vi "N8731ACTRL20.vi"() -> ()   [LabVIEW 2017]
uses:
  Controller subVIs/CurrentPSUSettings.vi
  Keysight N8731A conversion/Keysight N8900 Series.lvlib
panel:
  out "time":dbl
  out "I(t)":cluster{dbl[], dbl[]}(graph)
  out "V(t)":cluster{dbl[], dbl[]}(graph)
  in  "Sweep Controller":enum32{"Sweep Mode", "Free Control Mode"}(tab)=enum."Free Control Mode"
  in  "Voltage Limit [V]":dbl=8.0 min=0.0 max=8.0
  in  "Time Delay [s]":dbl=0.15
  in  "Step Size [A]":dbl=5.0 min=0.0 max=400.0
  in  "Start Current [A]":dbl min=0.0 max=400.0
  in  "End Current [A]":dbl=50.0 min=0.0 max=400.0
  out "Approx Sweep Time [min]":dbl
  in  "Start Voltage [V]":dbl min=0.0 max=8.0
  in  "Step Size [mV]":dbl=10.0 min=0.0
  in  "Current Limit [A]":dbl=150.0 min=0.0 max=400.0
  in  "End Voltage[V]":dbl=0.1 min=0.0 max=8.0
  in  "CC(1)/VC(0)":bool
  in  "Time between data points (ms)":i32=500 min=0
  in  "Sweepback Time (s)":dbl min=0.0
  out "Immediate Voltage (V)":dbl
  out "Immediate Current (A)":dbl
  in  "Voltage Set [V]":dbl min=0.0 max=8.0 step=0.001
  in  "Current Set [A]":dbl min=0.0 max=400.0 step=0.1
  out "Status message":string
  in  "Voltmeter channel (6)":i32=6
  in  "em. stop":bool
  in  "Stop Sweep":bool
  out "Voltmeter error message":errorcluster
  in  "Voltmeter Range (V)":dbl caption="0 for Auto range"
  in  "Voltmeter Address (16)":i16=16
  out "PSU error message":errorcluster
  in  "Start Sweep":bool
  in  "Sweepback":bool=TRUE
  in  "Power Output":bool
  in  "OC protection":bool
  in  "OV Value (10V)":dbl=10.0 min=0.5 max=10.0
  out "Sweeping Back":bool
  out "I(V) Graph":cluster{dbl[], dbl[]}(graph)
  in  "VISA resource name":refnum<visa-resource-name>="N8731APSU"
  in  "Filename":string caption="Leave empty to discard data.\nDon't touch during measurement"
  in  "PSU\nVoltage":bool=TRUE caption="Keithley\nVoltage"
  in  "OV protection":bool=TRUE
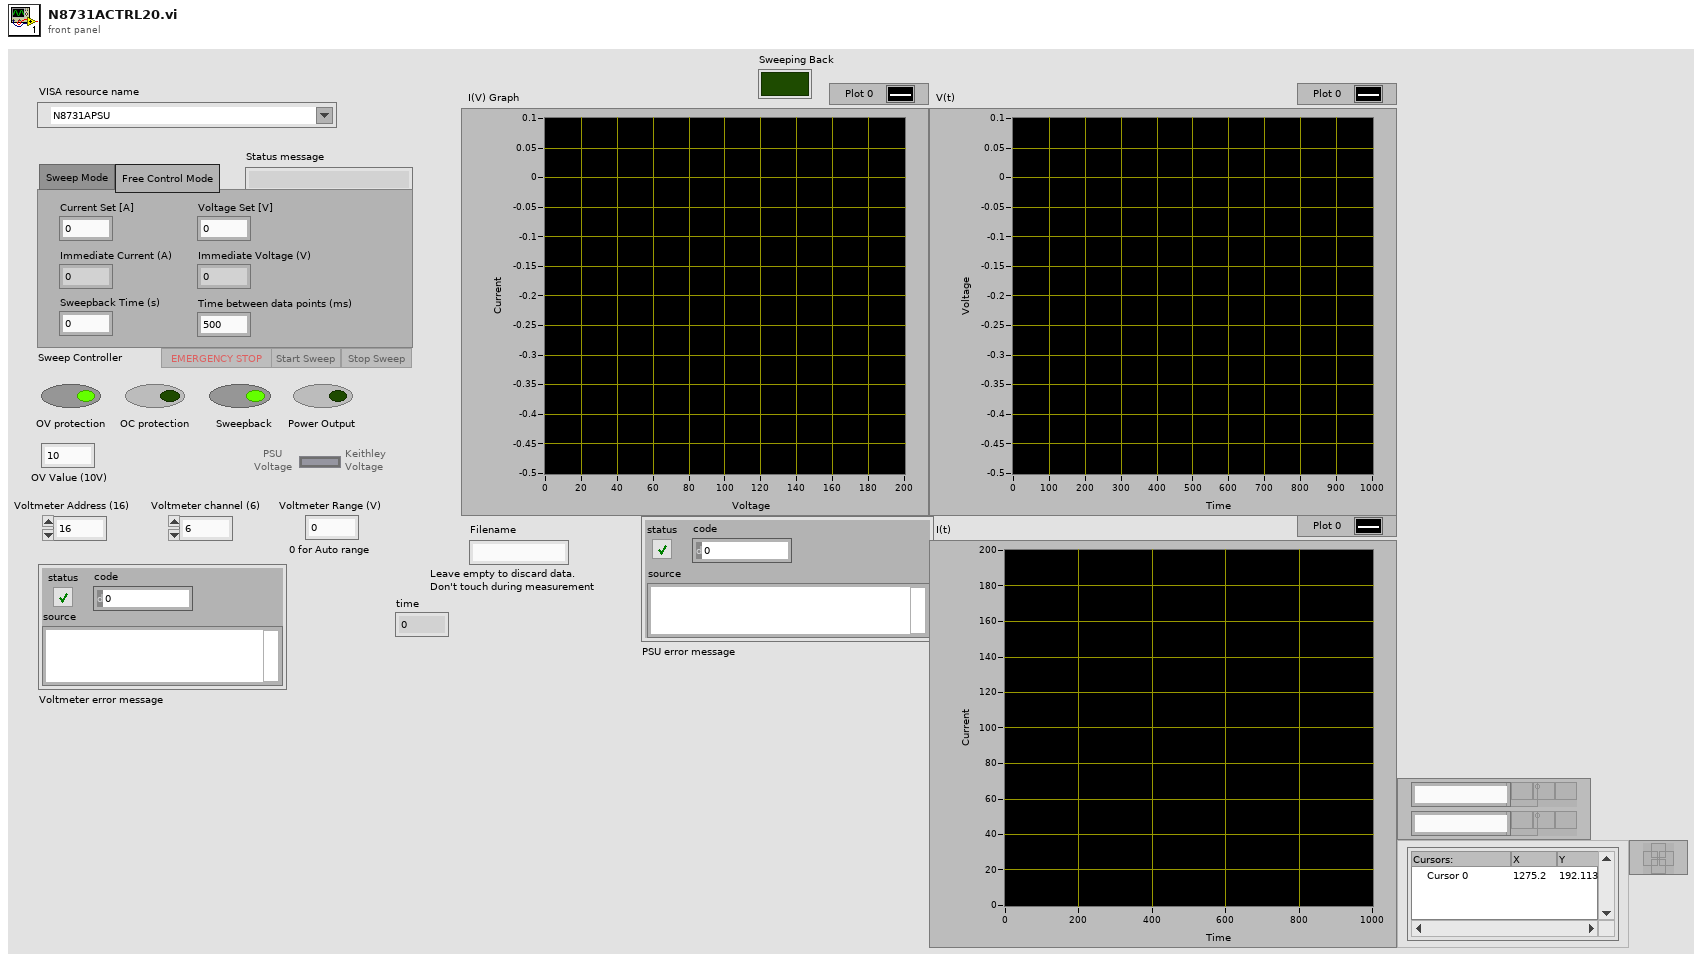
[diagram p1: front panel]
types:
  T1 = enum8{"Enabled", "Disabled", "Disabled and Grayed Out"}
  T2 = cluster{"CC(1)/VC(0)":bool, "Sweep Controller":enum32{"Sweep Mode", "Free Control Mode"}, "   PSU\nVoltage":bool}
  T3 = cluster{"CC(1)/VC(0)":bool, "Sweep Controller":bool, "   PSU\nVoltage":bool}
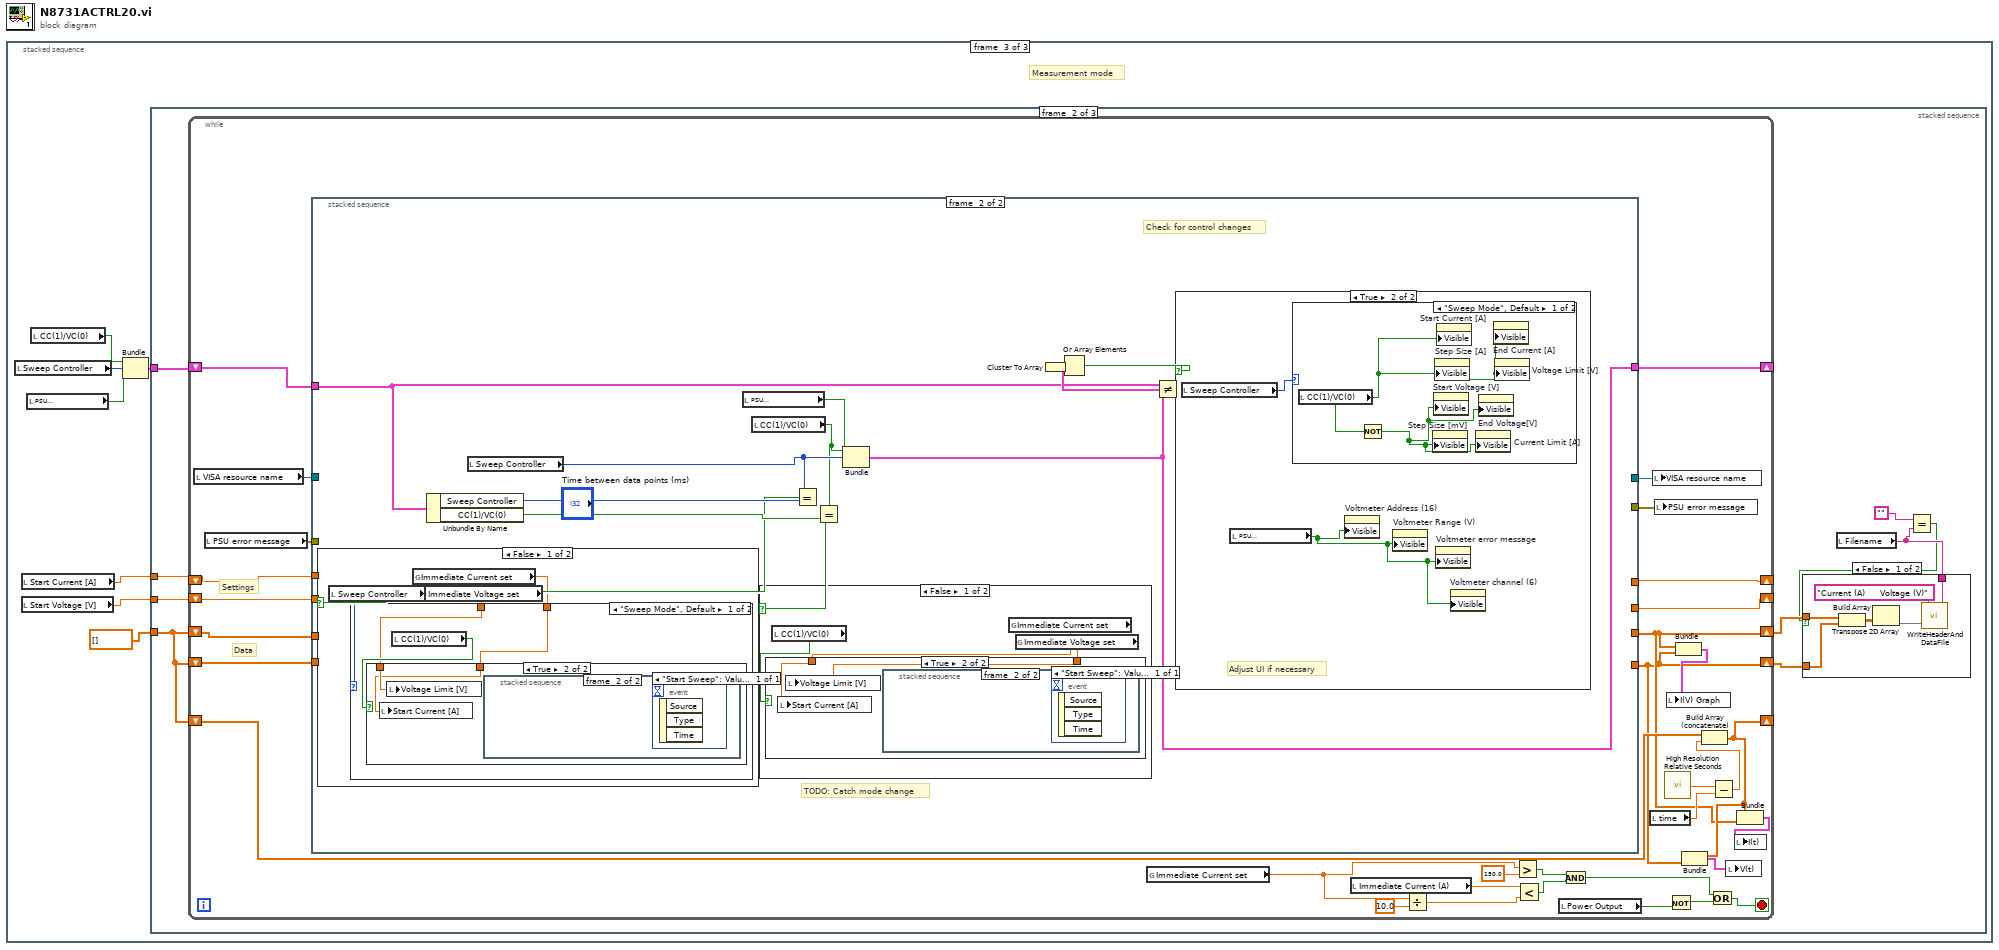
[diagram p0: block diagram]
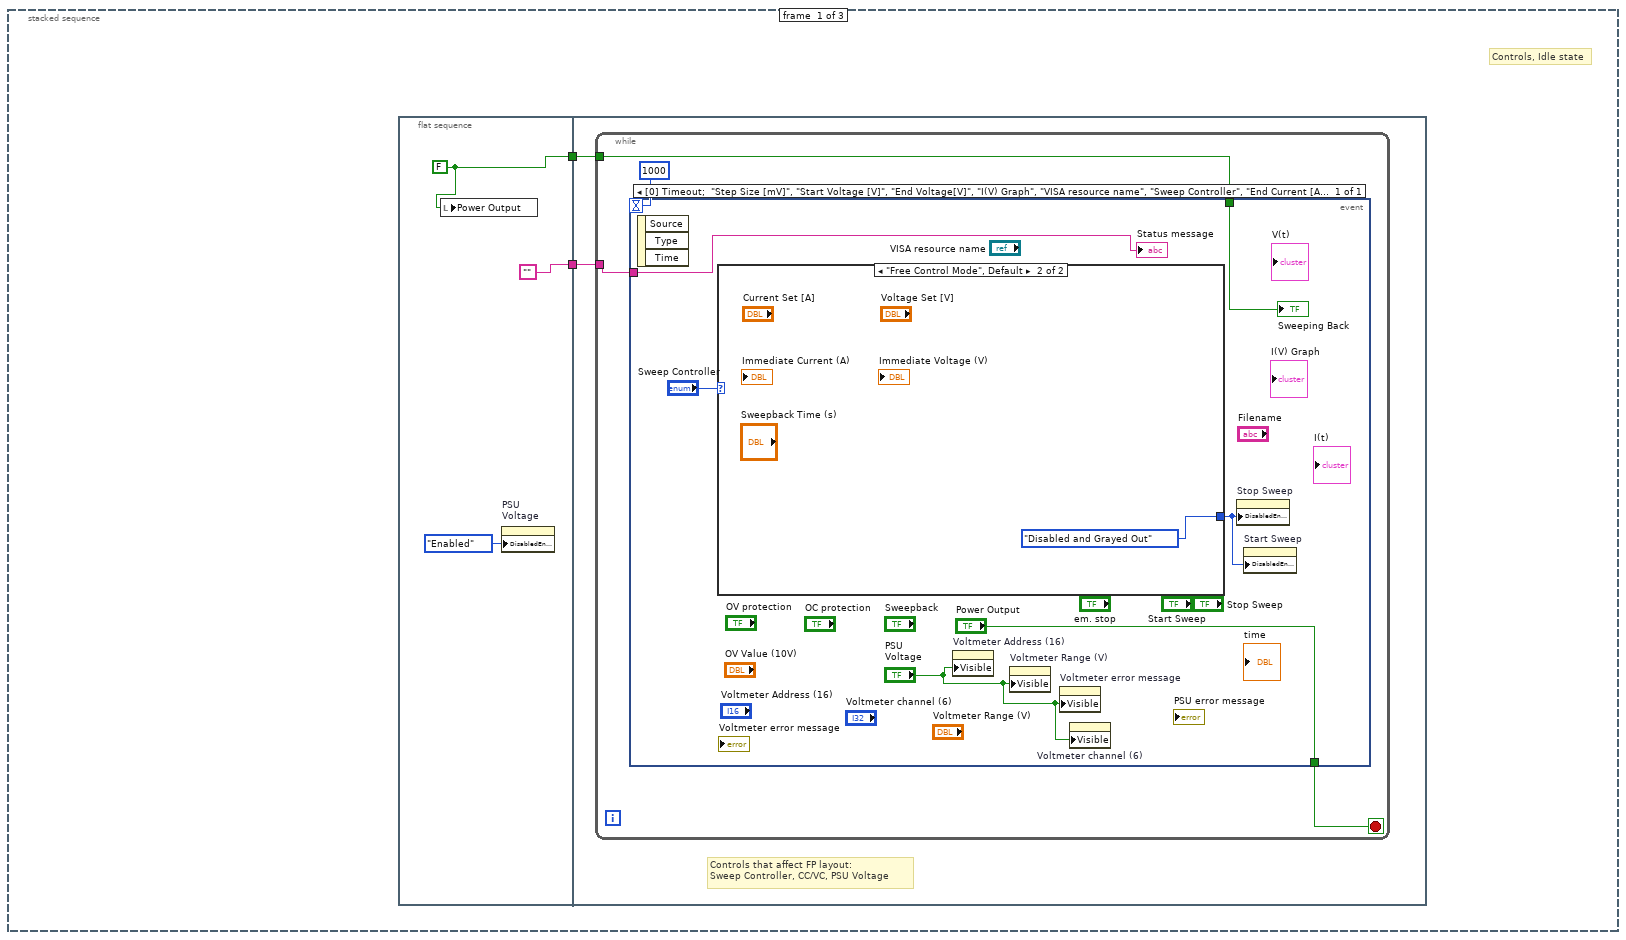
[diagram p2: hidden frame]
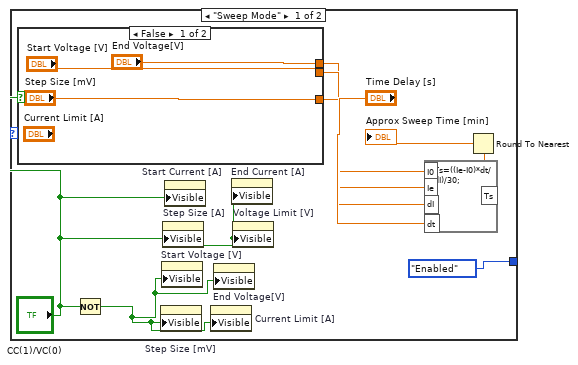
[diagram p3: hidden frame]
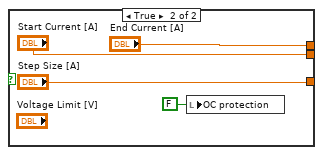
[diagram p4: hidden frame]
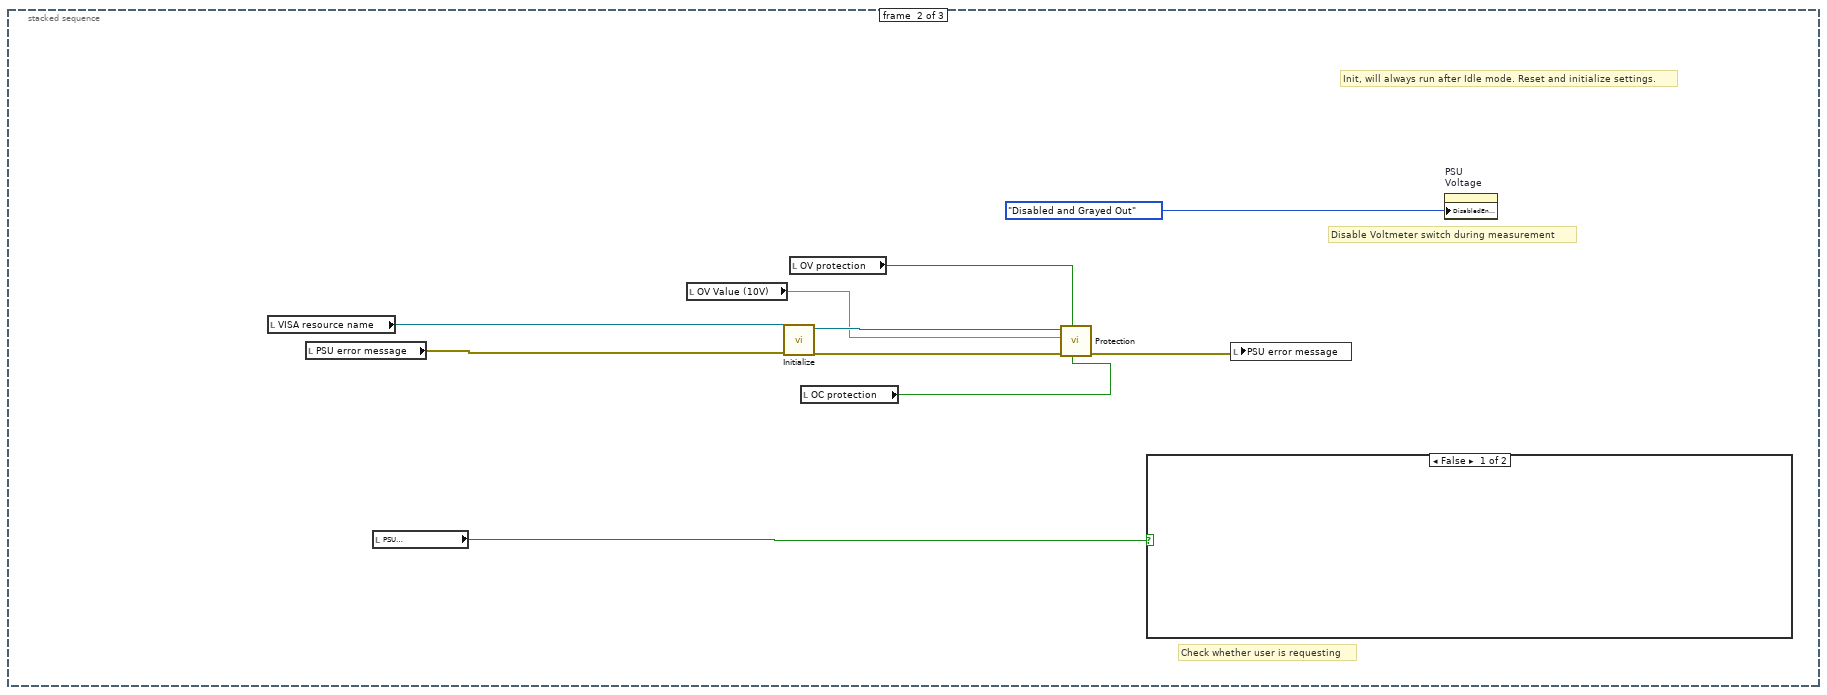
[diagram p5: hidden frame]
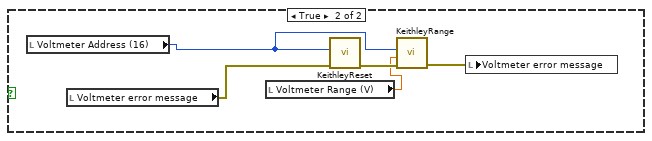
[diagram p6: hidden frame]
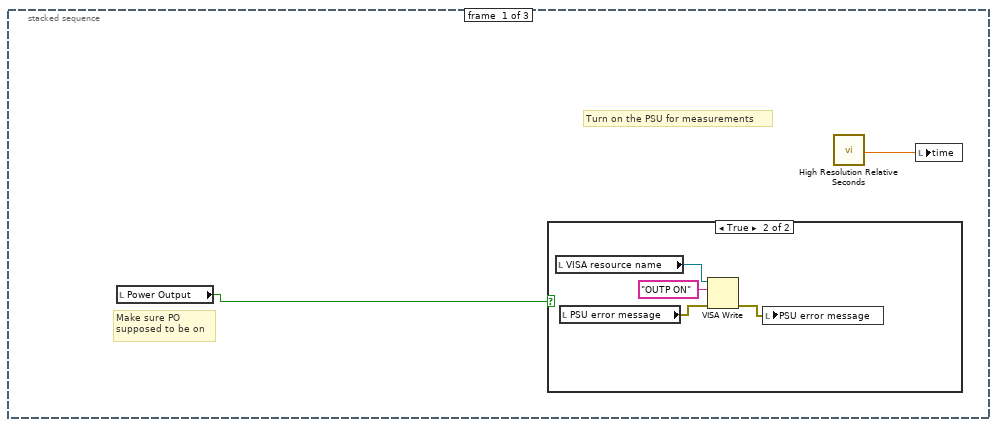
[diagram p7: hidden frame]
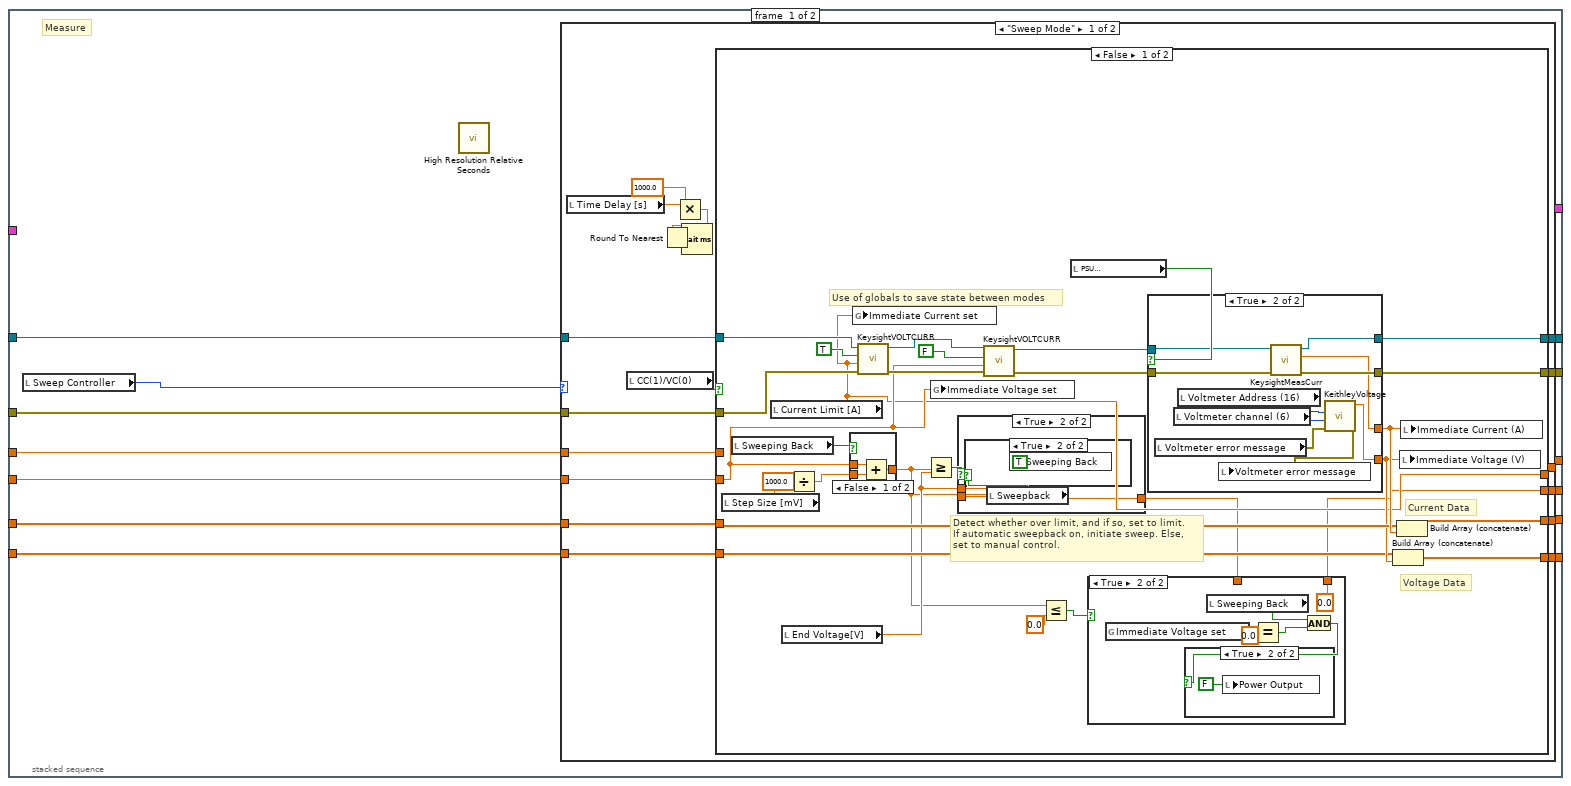
[diagram p10: hidden frame]
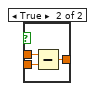
[diagram p13: hidden frame]
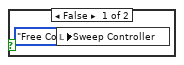
[diagram p15: hidden frame]
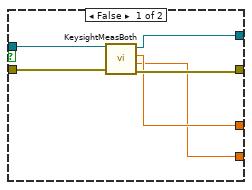
[diagram p16: hidden frame]
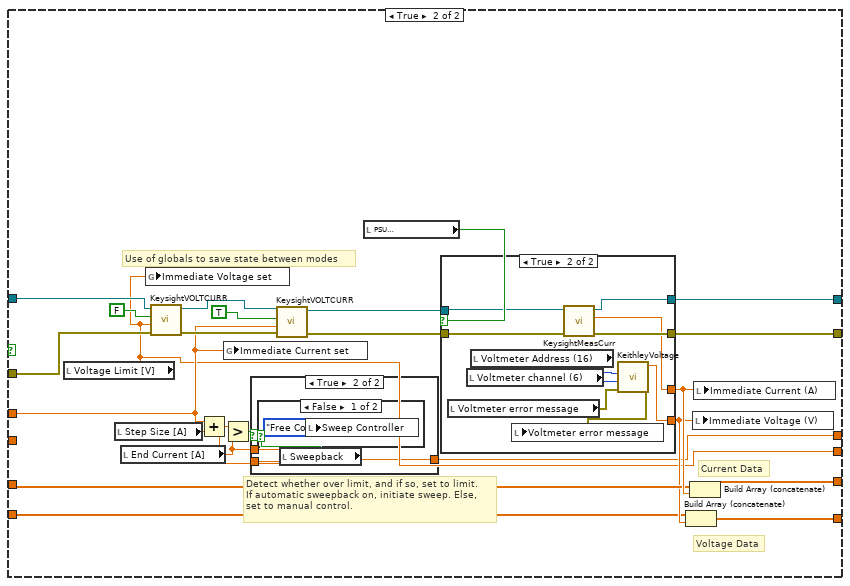
[diagram p17: hidden frame]
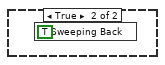
[diagram p19: hidden frame]
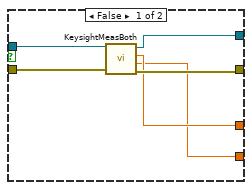
[diagram p20: hidden frame]
diagram:
  n1 = stacked-sequence {
    frame #0 {
      # "Controls, Idle state"
      n2 = flat-sequence {
        tunnel: [w3] -> w2
        tunnel: ["" ("Status message")] -> w1
        tunnel: w2 -> [w7]
        tunnel: w1 -> [w6]
        frame #0 {
          w3 = FALSE ("Sweeping Back")
          n3 = local write "Power Output"(w3) -> ()
          n4 = property on="PSU\nVoltage" class="Bool (strict)"("DisabledEnum"=T1."Enabled" ("Disabled")) -> ()  [unwired: 2 in, 2 out]
        }
        frame #1 {
          # "Controls that affect FP layout:\nSweep Controller, CC/VC, PSU Voltage"
          n5 = while {
            tunnel: w7 -> [w9]
            tunnel: w6 -> [w8]
            stop <- w11 stop-if-true
            n6 = event shown="[0] Timeout;  \"Step Size [mV]\", \"Start Voltage [V]\", \"End Voltage[V]\", \"I(V) Graph\", \"VISA resource name\", \"Sweep Controller\", \"End Current [A]\", \"Stop Sweep\", \"Start Current [A]\", \"Step Size [A]\", \"Time Delay [s]\", \"Current Limit [A]\", \"Voltage Limit [V]\", \"Approx Sweep Time [min]\", \"OV Value (10V)\", \"OC protection\", \"Sweeping Back\", \"Filename\", \"OV protection\", \"PSU Voltage\", \"CC(1)/VC(0)\": Value Change" {
              selector: _ -> [_]
              dyn-events: _ -> [_]
              timeout: 1000 -> [_]
              tunnel: ["Power Output"] -> w11
              tunnel: w9 -> [w14]
              tunnel: w8 -> [w12]
              event Timeout; "Step Size [mV]", "Start Voltage [V]", "End Voltage[V]", "I(V) Graph", "VISA resource name", "Sweep Controller", "End Current [A]", "Stop Sweep", "Start Current [A]", "Step Size [A]", "Time Delay [s]", "Current Limit [A]", "Voltage Limit [V]", "Approx Sweep Time [min]", "OV Value (10V)", "OC protection", "Sweeping Back", "Filename", "OV protection", "PSU\nVoltage", "CC(1)/VC(0)": Value Change {
                n7 = event-data() -> ()  [unwired: 1 in, 3 out]
                n8 = case shown="\"Free Control Mode\", Default" "Sweep Controller" {
                  tunnel: [T1."Enabled" ("Disabled") T1."Disabled and Grayed Out" ("Disabled")] -> w15
                  frame "Sweep Mode" {
                    n9 = case shown="False" "CC(1)/VC(0)" {
                      tunnel: ["Step Size [mV]" "Step Size [A]"] -> w25
                      tunnel: ["Start Voltage [V]" "Start Current [A]"] -> w22
                      tunnel: ["End Voltage[V]" "End Current [A]"] -> w21
                      frame False {
                      }
                      frame True {
                        n10 = local write "OC protection"(FALSE ("OC protection")) -> ()
                      }
                    }
                    n11 = Not(x="CC(1)/VC(0)") -> (.not. x?=w20:bool)
                    n12 = property on="Step Size [mV]" class="DigNum (strict)"("Visible"=w20) -> ()  [unwired: 2 in, 2 out]
                    n13 = property on="Start Voltage [V]" class="DigNum (strict)"("Visible"=w20) -> ()  [unwired: 2 in, 2 out]
                    n14 = property on="Step Size [A]" class="DigNum (strict)"("Visible"="CC(1)/VC(0)") -> ()  [unwired: 2 in, 2 out]
                    n15 = property on="Start Current [A]" class="DigNum (strict)"("Visible"="CC(1)/VC(0)") -> ()  [unwired: 2 in, 2 out]
                    n16 = property on="Current Limit [A]" class="DigNum (strict)"("Visible"=w20) -> ()  [unwired: 2 in, 2 out]
                    n17 = property on="End Voltage[V]" class="DigNum (strict)"("Visible"=w20) -> ()  [unwired: 2 in, 2 out]
                    n18 = property on="End Current [A]" class="DigNum (strict)"("Visible"="CC(1)/VC(0)") -> ()  [unwired: 2 in, 2 out]
                    n19 = property on="Voltage Limit [V]" class="DigNum (strict)"("Visible"="CC(1)/VC(0)") -> ()  [unwired: 2 in, 2 out]
                    n20 = formula code="Ts=((Ie-I0)*dt/dI)/30;"("I0"=w22, "Ie"=w21, "dI"=w25, "dt"="Time Delay [s]") -> ("Ts"=w24:dbl)
                    n21 = Round To Nearest(number=w24) -> (nearest integer value=→"Approx Sweep Time [min]":dbl)
                  }
                  frame "Free Control Mode", Default {
                  }
                }
                n22 = property on="Voltmeter Address (16)" class="DigNum (strict)"("Visible"="PSU\nVoltage") -> ()  [unwired: 2 in, 2 out]
                n23 = property on="Voltmeter Range (V)" class="DigNum (strict)"("Visible"="PSU\nVoltage") -> ()  [unwired: 2 in, 2 out]
                n24 = property on="Voltmeter error message" class="Clust (strict)"("Visible"="PSU\nVoltage") -> ()  [unwired: 2 in, 2 out]
                n25 = property on="Voltmeter channel (6)" class="DigNum (strict)"("Visible"="PSU\nVoltage") -> ()  [unwired: 2 in, 2 out]
                n26 = property on="Stop Sweep" class="Bool"("DisabledEnum"=w15) -> ()  [unwired: 2 in, 2 out]
                n27 = property on="Start Sweep" class="Bool"("DisabledEnum"=w15) -> ()  [unwired: 2 in, 2 out]
                "Sweeping Back" <- w14
                "Status message" <- w12
              }
            }
          }
        }
      }
    }
    frame #1 {
      # "Check whether user is requesting"
      # "Disable Voltmeter switch during measurement"
      # "Init, will always run after Idle mode. Reset and initialize settings."
      n28 = local read "VISA resource name"() -> (w42:refnum<visa-resource-name>)
      n29 = local read "PSU error message"() -> (w37:errorcluster)
      n30 = local read "PSU\nVoltage"() -> (w36:bool)
      n31 = local read "OV Value (10V)"() -> (w41:dbl)
      n32 = call "Initialize.vi"("error in (no error)"=w37, "VISA resource name"=w42) -> ("error out"=w43:errorcluster, "VISA resource name out"=w44:refnum<visa-resource-name>)  [unwired: 8 in]
      n33 = local read "OV protection"() -> (w39:bool)
      n34 = local read "OC protection"() -> (w40:bool)
      n35 = call "Protection.vi"("OC protection"=w40, "OV protection"=w39, "error in (no error)"=w43, "OV Value (10V)"=w41, "VISA resource name"=w44) -> ("error out"=w38:errorcluster)  [unwired: 5 in, 1 out]
      n36 = case shown="False" w36 {
        frame False {
        }
        frame True {
          n37 = local read "Voltmeter Address (16)"() -> (w45:i16)
          n38 = local read "Voltmeter error message"() -> (w47:errorcluster)
          n39 = local read "Voltmeter Range (V)"() -> (w46:dbl)
          n40 = call "KeithleyReset.vi"("error in"=w47, "address (16)"=w45) -> ("error out"=w48:errorcluster)  [unwired: 9 in]
          n41 = call "KeithleyRange.vi"("error in"=w48, "Range (V)/Auto(0)"=w46, "address (16)"=w45) -> ("error out"=w49:errorcluster)  [unwired: 8 in]
          n42 = local write "Voltmeter error message"(w49) -> ()
        }
      }
      n43 = local write "PSU error message"(w38) -> ()
      n44 = property on="PSU\nVoltage" class="Bool (strict)"("DisabledEnum"=T1."Disabled and Grayed Out" ("Disabled")) -> ()  [unwired: 2 in, 2 out]
    }
    frame #2 {
      # "Measurement mode"
      n45 = local read "Sweep Controller"() -> (w55:enum32{"Sweep Mode", "Free Control Mode"})
      n46 = local read "Start Current [A]"() -> (w52:dbl)
      n47 = local read "Start Voltage [V]"() -> (w51:dbl)
      n48 = local read "PSU\nVoltage"() -> (w54:bool)
      n49 = local read "CC(1)/VC(0)"() -> (w56:bool)
      n50 = Bundle("CC(1)/VC(0)"=w56, "Sweep Controller"=w55, "PSU\nVoltage"=w54) -> (w53:T2)  [unwired: 1 in]
      n51 = stacked-sequence {
        tunnel: w53 -> [_ w71 _]
        tunnel: w52 -> [_ w70 _]
        tunnel: w51 -> [_ w69 _]
        tunnel: dbl[] [] -> [_ w63 _]
        frame #0 {
          # "Make sure PO\nsupposed to be on"
          # "Turn on the PSU for measurements"
          n52 = local read "Power Output"() -> (w58:bool)
          n53 = case shown="True" w58 {
            frame False {
            }
            frame True {
              n54 = local read "VISA resource name"() -> (w61:refnum<visa-resource-name>)
              n55 = local read "PSU error message"() -> (w60:errorcluster)
              n56 = VISA Write(VISA resource name=w61, write buffer="OUTP ON", error in (no error)=w60) -> (error out=w59:errorcluster)  [unwired: 2 out]
              n57 = local write "PSU error message"(w59) -> ()
            }
          }
          n58 = call <vilib>:"High Resolution Relative Seconds.vi"() -> ("relative seconds"=w57:dbl)
          n59 = local write "time"(w57) -> ()
        }
        frame #1 {
          n60 = while {
            shift-right: [w109] -> _
            shift-left: w71 -> [w110]
            shift-right: [w100] -> _
            shift-left: w69 -> [w98]
            shift-right: [w101] -> _
            shift-left: w70 -> [w106]
            shift-right: [w91] -> w68
            shift-left: w63 -> [w103]
            shift-right: [w90] -> w67
            shift-left: w63 -> [w102]
            shift-right: [w92] -> _
            shift-left: w63 -> [w96]
            stop <- w78 stop-if-true
            # "Data"
            # "Settings"
            n61 = local read "VISA resource name"() -> (w108:refnum<visa-resource-name>)
            n62 = local read "PSU error message"() -> (w107:errorcluster)
            n63 = stacked-sequence {
              tunnel: w110 -> [_ w295]
              tunnel: [_ w299] -> w109
              tunnel: w108 -> [w122 _]
              tunnel: w107 -> [w121 _]
              tunnel: w106 -> [w120 _]
              tunnel: [w119 _] -> w105
              tunnel: [w118 _] -> w104
              tunnel: w103 -> [w117 _]
              tunnel: [w116 _] -> w91
              tunnel: w102 -> [w115 _]
              tunnel: [w114 _] -> w90
              tunnel: [w113 _] -> w101
              tunnel: [w112 _] -> w100
              tunnel: w98 -> [w111 _]
              frame #0 {
                # "Measure"
                n64 = local read "Sweep Controller"() -> (w123:enum32{"Sweep Mode", "Free Control Mode"})
                n65 = call <vilib>:"High Resolution Relative Seconds.vi"() -> ()  [unwired: 1 out]
                n66 = case shown="\"Sweep Mode\"" w123 {
                  tunnel: w122 -> [w139 w272]
                  tunnel: w121 -> [w138 w271]
                  tunnel: w120 -> [w137 _]
                  tunnel: [w136 w270] -> w119
                  tunnel: [w135 w269] -> w118
                  tunnel: w117 -> [w134 w268]
                  tunnel: [w133 w267] -> w116
                  tunnel: w115 -> [w132 w266]
                  tunnel: [w131 w265] -> w114
                  tunnel: [w130 w253] -> w113
                  tunnel: [w129 w252] -> w112
                  tunnel: w111 -> [w128 _]
                  frame "Sweep Mode" {
                    n67 = local read "Time Delay [s]"() -> (w127:dbl)
                    n68 = local read "CC(1)/VC(0)"() -> (w140:bool)
                    n69 = Multiply(x=w127, y=1000.0) -> (x*y=w125:dbl)
                    n70 = Round To Nearest(number=w125) -> (nearest integer value=w124:dbl)
                    n71 = Wait (ms)(milliseconds to wait=w124) -> ()  [unwired: 1 out]
                    n72 = case shown="False" w140 {
                      tunnel: w139 -> [w166 w225]
                      tunnel: w138 -> [w165 w224]
                      tunnel: w137 -> [_ w223]
                      tunnel: [w161 w218] -> w136
                      tunnel: [w160 w217] -> w135
                      tunnel: w134 -> [w158 w215]
                      tunnel: [w149 w214] -> w133
                      tunnel: w132 -> [w156 w212]
                      tunnel: [w155 w211] -> w131
                      tunnel: [w148 w209] -> w130
                      tunnel: [w142 w210] -> w129
                      tunnel: w128 -> [w150 _]
                      frame False {
                        # "Use of globals to save state between modes"
                        # "Detect whether over limit, and if so, set to limit.\nIf automatic sweepback on, initiate sweep. Else,\nset to manual control."
                        # "Voltage Data"
                        # "Current Data"
                        n73 = local read "Step Size [mV]"() -> (w153:dbl)
                        n74 = local read "Sweeping Back"() -> (w146:bool)
                        n75 = local read "Current Limit [A]"() -> (w148:dbl)
                        n76 = local read "End Voltage[V]"() -> (w147:dbl)
                        n77 = Divide(x=w153, y=1000.0) -> (x/y=w152:dbl)
                        n78 = case shown="False" w146 {
                          tunnel: [w181 w182] -> w144
                          tunnel: w152 -> [w180 w184]
                          tunnel: w150 -> [w179 w183]
                          frame False {
                            n79 = Add(x=w179, y=w180) -> (x+y=w181:dbl)
                          }
                          frame True {
                            n80 = Subtract(x=w183, y=w184) -> (x-y=w182:dbl)
                          }
                        }
                        n81 = global write "CurrentPSUSettings.vi" "Immediate Current set"(w148) -> ()
                        n82 = call "KeysightVOLTCURR.vi"("error in (no error)"=w165, "CURR/VOLT (A/V)"=w148, "CURR (1)/VOLT (0)"=TRUE, "VISA resource name"=w166) -> ("error out"=w167:errorcluster, "VISA resource name out"=w168:refnum<visa-resource-name>)  [unwired: 6 in]
                        n83 = Greater Or Equal?(x=w144, y=w147) -> (x >= y?=w154:bool)
                        n84 = global write "CurrentPSUSettings.vi" "Immediate Voltage set"(w150) -> ()
                        n85 = case shown="True" w154 {
                          tunnel: w144 -> [w185 _]
                          tunnel: [w185 w187] -> w143
                          tunnel: w147 -> [_ w187]
                          frame False {
                          }
                          frame True {
                            n86 = local read "Sweepback"() -> (w186:bool)
                            n87 = case shown="True" w186 {
                              frame False {
                                n88 = local write "Sweep Controller"(enum32{"Sweep Mode", "Free Control Mode"}."Free Control Mode" ("Sweep Controller")) -> ()
                              }
                              frame True {
                                n89 = local write "Sweeping Back"(TRUE ("Sweeping Back")) -> ()
                              }
                            }
                          }
                        }
                        n90 = call "KeysightVOLTCURR.vi"("error in (no error)"=w167, "CURR/VOLT (A/V)"=w150, "CURR (1)/VOLT (0)"=FALSE, "VISA resource name"=w168) -> ("error out"=w162:errorcluster, "VISA resource name out"=w163:refnum<visa-resource-name>)  [unwired: 6 in]
                        n91 = Less Or Equal?(x=w144, y=0.0) -> (x <= y?=w141:bool)
                        n92 = local read "PSU\nVoltage"() -> (w164:bool)
                        n93 = case shown="True" w141 {
                          tunnel: w143 -> [w171 _]
                          tunnel: [w171 0.0 ("End Voltage[V]")] -> w142
                          frame False {
                          }
                          frame True {
                            n94 = global read "CurrentPSUSettings.vi" "Immediate Voltage set"() -> (w175:dbl)
                            n95 = local read "Sweeping Back"() -> (w176:bool)
                            n96 = Equal?(x=w175, y=0.0) -> (x = y?=w173:bool)
                            n97 = And(x=w176, y=w173) -> (x .and. y?=w172:bool)
                            n98 = case shown="True" w172 {
                              frame False {
                              }
                              frame True {
                                n99 = local write "Power Output"(FALSE ("Power Output")) -> ()
                              }
                            }
                          }
                        }
                        n100 = case shown="True" w164 {
                          tunnel: w163 -> [w195 w205]
                          tunnel: w162 -> [w194 w204]
                          tunnel: [w193 w199] -> w161
                          tunnel: [w192 w198] -> w160
                          tunnel: [w191 w197] -> w159
                          tunnel: [w190 w196] -> w157
                          frame False {
                            n101 = call "KeysightMeasBoth.vi"("error in (no error)"=w194, "VISA resource name"=w195) -> ("error out"=w192:errorcluster, "VOLT"=w190:dbl, "CURR"=w191:dbl, "VISA resource name out"=w193:refnum<visa-resource-name>)  [unwired: 6 in]
                          }
                          frame True {
                            n102 = local read "Voltmeter error message"() -> (w201:errorcluster)
                            n103 = local read "Voltmeter channel (6)"() -> (w203:i32)
                            n104 = local read "Voltmeter Address (16)"() -> (w202:i16)
                            n105 = call "KeysightMeasCurr.vi"("error in (no error)"=w204, "VISA resource name"=w205) -> ("error out"=w198:errorcluster, "CURR"=w197:dbl, "VISA resource name out"=w199:refnum<visa-resource-name>)  [unwired: 7 in]
                            n106 = call "KeithleyVoltage.vi"("error in"=w201, "channel (6)"=w203, "address (16)"=w202) -> ("error out"=w200:errorcluster, "Voltage"=w196:dbl)  [unwired: 7 in]
                            n107 = local write "Voltmeter error message"(w200) -> ()
                          }
                        }
                        n108 = Build Array (concatenate)(w156, w157) -> (w155:dbl[])
                        n109 = Build Array (concatenate)(w158, w159) -> (w149:dbl[])
                        n110 = local write "Immediate Voltage (V)"(w157) -> ()
                        n111 = local write "Immediate Current (A)"(w159) -> ()
                      }
                      frame True {
                        # "Use of globals to save state between modes"
                        # "Detect whether over limit, and if so, set to limit.\nIf automatic sweepback on, initiate sweep. Else,\nset to manual control."
                        # "Voltage Data"
                        # "Current Data"
                        n112 = local read "Voltage Limit [V]"() -> (w210:dbl)
                        n113 = local read "Step Size [A]"() -> (w222:dbl)
                        n114 = local read "End Current [A]"() -> (w206:dbl)
                        n115 = global write "CurrentPSUSettings.vi" "Immediate Voltage set"(w210) -> ()
                        n116 = call "KeysightVOLTCURR.vi"("error in (no error)"=w224, "CURR/VOLT (A/V)"=w210, "CURR (1)/VOLT (0)"=FALSE, "VISA resource name"=w225) -> ("error out"=w226:errorcluster, "VISA resource name out"=w227:refnum<visa-resource-name>)  [unwired: 6 in]
                        n117 = Add(x=w223, y=w222) -> (x+y=w207:dbl)
                        n118 = Greater?(x=w207, y=w206) -> (0:w208:bool)
                        n119 = global write "CurrentPSUSettings.vi" "Immediate Current set"(w223) -> ()
                        n120 = case shown="True" w208 {
                          tunnel: w207 -> [w230 _]
                          tunnel: [w230 w232] -> w209
                          tunnel: w206 -> [_ w232]
                          frame False {
                          }
                          frame True {
                            n121 = local read "Sweepback"() -> (w231:bool)
                            n122 = case shown="False" w231 {
                              frame False {
                                n123 = local write "Sweep Controller"(enum32{"Sweep Mode", "Free Control Mode"}."Free Control Mode" ("Sweep Controller")) -> ()
                              }
                              frame True {
                                n124 = local write "Sweeping Back"(TRUE ("Sweeping Back")) -> ()
                              }
                            }
                          }
                        }
                        n125 = call "KeysightVOLTCURR.vi"("error in (no error)"=w226, "CURR/VOLT (A/V)"=w223, "CURR (1)/VOLT (0)"=TRUE, "VISA resource name"=w227) -> ("error out"=w219:errorcluster, "VISA resource name out"=w220:refnum<visa-resource-name>)  [unwired: 6 in]
                        n126 = local read "PSU\nVoltage"() -> (w221:bool)
                        n127 = case shown="True" w221 {
                          tunnel: w220 -> [w240 w250]
                          tunnel: w219 -> [w239 w249]
                          tunnel: [w238 w244] -> w218
                          tunnel: [w237 w243] -> w217
                          tunnel: [w236 w242] -> w216
                          tunnel: [w235 w241] -> w213
                          frame False {
                            n128 = call "KeysightMeasBoth.vi"("error in (no error)"=w239, "VISA resource name"=w240) -> ("error out"=w237:errorcluster, "VOLT"=w235:dbl, "CURR"=w236:dbl, "VISA resource name out"=w238:refnum<visa-resource-name>)  [unwired: 6 in]
                          }
                          frame True {
                            n129 = local read "Voltmeter error message"() -> (w246:errorcluster)
                            n130 = local read "Voltmeter channel (6)"() -> (w248:i32)
                            n131 = local read "Voltmeter Address (16)"() -> (w247:i16)
                            n132 = call "KeysightMeasCurr.vi"("error in (no error)"=w249, "VISA resource name"=w250) -> ("error out"=w243:errorcluster, "CURR"=w242:dbl, "VISA resource name out"=w244:refnum<visa-resource-name>)  [unwired: 7 in]
                            n133 = call "KeithleyVoltage.vi"("error in"=w246, "channel (6)"=w248, "address (16)"=w247) -> ("error out"=w245:errorcluster, "Voltage"=w241:dbl)  [unwired: 7 in]
                            n134 = local write "Voltmeter error message"(w245) -> ()
                          }
                        }
                        n135 = Build Array (concatenate)(w212, w213) -> (w211:dbl[])
                        n136 = Build Array (concatenate)(w215, w216) -> (w214:dbl[])
                        n137 = local write "Immediate Voltage (V)"(w213) -> ()
                        n138 = local write "Immediate Current (A)"(w216) -> ()
                      }
                    }
                  }
                  frame "Free Control Mode", Default {
                    # "Use of globals to save state between modes"
                    # "Detect whether over limit, and if so, set to limit.\nIf automatic sweepback on, initiate sweep. Else,\nset to manual control."
                    # "Voltage Data"
                    # "Current Data"
                    n139 = local read "Time between data points (ms)"() -> (w251:i32)
                    n140 = local read "Current Set [A]"() -> (w264:dbl)
                    n141 = Wait (ms)(milliseconds to wait=w251) -> ()  [unwired: 1 out]
                    n142 = local read "Voltage Set [V]"() -> (w255:dbl)
                    n143 = global write "CurrentPSUSettings.vi" "Immediate Current set"(w264) -> ()
                    n144 = call "KeysightVOLTCURR.vi"("error in (no error)"=w271, "CURR/VOLT (A/V)"=w264, "CURR (1)/VOLT (0)"=TRUE, "VISA resource name"=w272) -> ("error out"=w260:errorcluster, "VISA resource name out"=w261:refnum<visa-resource-name>)  [unwired: 6 in]
                    n145 = global write "CurrentPSUSettings.vi" "Immediate Voltage set"(w255) -> ()
                    n146 = call "KeysightVOLTCURR.vi"("error in (no error)"=w260, "CURR/VOLT (A/V)"=w255, "CURR (1)/VOLT (0)"=FALSE, "VISA resource name"=w261) -> ("error out"=w257:errorcluster, "VISA resource name out"=w258:refnum<visa-resource-name>)  [unwired: 6 in]
                    n147 = local read "PSU\nVoltage"() -> (w259:bool)
                    n148 = case shown="True" w259 {
                      tunnel: w258 -> [w278 w288]
                      tunnel: w257 -> [w277 w287]
                      tunnel: [w276 w282] -> w270
                      tunnel: [w275 w281] -> w269
                      tunnel: [w274 w280] -> w256
                      tunnel: [w273 w279] -> w254
                      frame False {
                        n149 = call "KeysightMeasBoth.vi"("error in (no error)"=w277, "VISA resource name"=w278) -> ("error out"=w275:errorcluster, "VOLT"=w273:dbl, "CURR"=w274:dbl, "VISA resource name out"=w276:refnum<visa-resource-name>)  [unwired: 6 in]
                      }
                      frame True {
                        n150 = local read "Voltmeter error message"() -> (w284:errorcluster)
                        n151 = local read "Voltmeter channel (6)"() -> (w286:i32)
                        n152 = local read "Voltmeter Address (16)"() -> (w285:i16)
                        n153 = call "KeysightMeasCurr.vi"("error in (no error)"=w287, "VISA resource name"=w288) -> ("error out"=w281:errorcluster, "CURR"=w280:dbl, "VISA resource name out"=w282:refnum<visa-resource-name>)  [unwired: 7 in]
                        n154 = call "KeithleyVoltage.vi"("error in"=w284, "channel (6)"=w286, "address (16)"=w285) -> ("error out"=w283:errorcluster, "Voltage"=w279:dbl)  [unwired: 7 in]
                        n155 = local write "Voltmeter error message"(w283) -> ()
                      }
                    }
                    n156 = local write "Immediate Voltage (V)"(w254) -> ()
                    n157 = Build Array (concatenate)(w266, w254) -> (w265:dbl[])
                    n158 = global read "CurrentPSUSettings.vi" "Immediate Current set"() -> (w253:dbl)
                    n159 = global read "CurrentPSUSettings.vi" "Immediate Voltage set"() -> (w252:dbl)
                    n160 = Build Array (concatenate)(w268, w256) -> (w267:dbl[])
                    n161 = local write "Immediate Current (A)"(w256) -> ()
                  }
                }
              }
              frame #1 {
                # "TODO: Catch mode change"
                # "Check for control changes"
                n162 = Unbundle By Name(w295) -> ("Sweep Controller"=w293:enum32{"Sweep Mode", "Free Control Mode"}, "CC(1)/VC(0)"=w292:bool)
                n163 = local read "Sweep Controller"() -> (w294:enum32{"Sweep Mode", "Free Control Mode"})
                n164 = local read "PSU\nVoltage"() -> (w300:bool)
                n165 = local read "CC(1)/VC(0)"() -> (w291:bool)
                n166 = Equal?(x=w294, y=w293) -> (x = y?=w290:bool)
                n167 = case shown="False" w290 {
                  frame False {
                    n168 = local read "Sweep Controller"() -> (w312:enum32{"Sweep Mode", "Free Control Mode"})
                    n169 = global read "CurrentPSUSettings.vi" "Immediate Current set"() -> (w310:dbl)
                    n170 = global read "CurrentPSUSettings.vi" "Immediate Voltage set"() -> (w311:dbl)
                    n171 = case shown="\"Sweep Mode\", Default" w312 {
                      tunnel: w311 -> [w314 w323]
                      tunnel: w310 -> [w313 w322]
                      frame "Sweep Mode", Default {
                        n172 = local read "CC(1)/VC(0)"() -> (w315:bool)
                        n173 = case shown="True" w315 {
                          tunnel: w314 -> [w317 w320]
                          tunnel: w313 -> [w316 w319]
                          frame False {
                            n174 = local write "Start Voltage [V]"(w317) -> ()
                            n175 = local write "Current Limit [A]"(w316) -> ()
                            n176 = stacked-sequence {
                              frame #0 {
                                n177 = local write "Status message"("Awaiting sweep confirmation" ("Status message")) -> ()
                              }
                              frame #1 {
                                n178 = event shown="[0] \"Start Sweep\": Value Change" {
                                selector: _ -> [_]
                                dyn-events: _ -> [_]
                                timeout: _ -> [_]
                                event "Start Sweep": Value Change {
                                n179 = event-data() -> ()  [unwired: 1 in, 3 out]
                                }
                                }
                              }
                            }
                          }
                          frame True {
                            n180 = local write "Start Current [A]"(w319) -> ()
                            n181 = local write "Voltage Limit [V]"(w320) -> ()
                            n182 = stacked-sequence {
                              frame #0 {
                                n183 = local write "Status message"("Awaiting sweep confirmation" ("Status message")) -> ()
                              }
                              frame #1 {
                                n184 = event shown="[0] \"Start Sweep\": Value Change" {
                                selector: _ -> [_]
                                dyn-events: _ -> [_]
                                timeout: _ -> [_]
                                event "Start Sweep": Value Change {
                                n185 = event-data() -> ()  [unwired: 1 in, 3 out]
                                }
                                }
                              }
                            }
                          }
                        }
                      }
                      frame "Free Control Mode" {
                        n186 = local write "Voltage Set [V]"(w323) -> ()
                        n187 = local write "Current Set [A]"(w322) -> ()
                      }
                    }
                  }
                  frame True {
                  }
                }
                n188 = Equal?(x=w291, y=w292) -> (x = y?=w289:bool)
                n189 = case shown="False" w289 {
                  frame False {
                    n190 = local read "CC(1)/VC(0)"() -> (w303:bool)
                    n191 = global read "CurrentPSUSettings.vi" "Immediate Current set"() -> (w301:dbl)
                    n192 = global read "CurrentPSUSettings.vi" "Immediate Voltage set"() -> (w302:dbl)
                    n193 = case shown="True" w303 {
                      tunnel: w302 -> [w305 w308]
                      tunnel: w301 -> [w304 w307]
                      frame False {
                        n194 = local write "Start Voltage [V]"(w305) -> ()
                        n195 = local write "Current Limit [A]"(w304) -> ()
                        n196 = stacked-sequence {
                          frame #0 {
                            n197 = local write "Status message"("Awaiting sweep confirmation" ("Status message")) -> ()
                          }
                          frame #1 {
                            n198 = event shown="[0] \"Start Sweep\": Value Change" {
                              selector: _ -> [_]
                              dyn-events: _ -> [_]
                              timeout: _ -> [_]
                              event "Start Sweep": Value Change {
                                n199 = event-data() -> ()  [unwired: 1 in, 3 out]
                              }
                            }
                          }
                        }
                      }
                      frame True {
                        n200 = local write "Start Current [A]"(w307) -> ()
                        n201 = local write "Voltage Limit [V]"(w308) -> ()
                        n202 = stacked-sequence {
                          frame #0 {
                            n203 = local write "Status message"("Awaiting sweep confirmation" ("Status message")) -> ()
                          }
                          frame #1 {
                            n204 = event shown="[0] \"Start Sweep\": Value Change" {
                              selector: _ -> [_]
                              dyn-events: _ -> [_]
                              timeout: _ -> [_]
                              event "Start Sweep": Value Change {
                                n205 = event-data() -> ()  [unwired: 1 in, 3 out]
                              }
                            }
                          }
                        }
                      }
                    }
                  }
                  frame True {
                  }
                }
                n206 = Bundle("CC(1)/VC(0)"=w291, "Sweep Controller"=w294, "PSU\nVoltage"=w300) -> (w299:T2)  [unwired: 1 in]
                n207 = Not Equal?(x=w295, y=w299) -> (x != y?=w298:T3)
                n208 = Cluster To Array(cluster=w298) -> (array=w297:bool[])
                n209 = Or Array Elements(Boolean array=w297) -> (logical OR=w296:bool)
                n210 = case shown="True" w296 {
                  frame False {
                  }
                  frame True {
                    # "Adjust UI if necessary"
                    n211 = local read "Sweep Controller"() -> (w325:enum32{"Sweep Mode", "Free Control Mode"})
                    n212 = local read "PSU\nVoltage"() -> (w324:bool)
                    n213 = case shown="\"Sweep Mode\", Default" w325 {
                      frame "Sweep Mode", Default {
                        n214 = local read "CC(1)/VC(0)"() -> (w326:bool)
                        n215 = Not(x=w326) -> (.not. x?=w327:bool)
                        n216 = property on="Step Size [mV]" class="DigNum (strict)"("Visible"=w327) -> ()  [unwired: 2 in, 2 out]
                        n217 = property on="Start Voltage [V]" class="DigNum (strict)"("Visible"=w327) -> ()  [unwired: 2 in, 2 out]
                        n218 = property on="Step Size [A]" class="DigNum (strict)"("Visible"=w326) -> ()  [unwired: 2 in, 2 out]
                        n219 = property on="Start Current [A]" class="DigNum (strict)"("Visible"=w326) -> ()  [unwired: 2 in, 2 out]
                        n220 = property on="Current Limit [A]" class="DigNum (strict)"("Visible"=w327) -> ()  [unwired: 2 in, 2 out]
                        n221 = property on="End Voltage[V]" class="DigNum (strict)"("Visible"=w327) -> ()  [unwired: 2 in, 2 out]
                        n222 = property on="End Current [A]" class="DigNum (strict)"("Visible"=w326) -> ()  [unwired: 2 in, 2 out]
                        n223 = property on="Voltage Limit [V]" class="DigNum (strict)"("Visible"=w326) -> ()  [unwired: 2 in, 2 out]
                      }
                      frame "Free Control Mode" {
                      }
                    }
                    n224 = property on="Voltmeter Address (16)" class="DigNum (strict)"("Visible"=w324) -> ()  [unwired: 2 in, 2 out]
                    n225 = property on="Voltmeter Range (V)" class="DigNum (strict)"("Visible"=w324) -> ()  [unwired: 2 in, 2 out]
                    n226 = property on="Voltmeter error message" class="Clust (strict)"("Visible"=w324) -> ()  [unwired: 2 in, 2 out]
                    n227 = property on="Voltmeter channel (6)" class="DigNum (strict)"("Visible"=w324) -> ()  [unwired: 2 in, 2 out]
                  }
                }
              }
            }
            n228 = global read "CurrentPSUSettings.vi" "Immediate Current set"() -> (w83:dbl)
            n229 = local read "Immediate Current (A)"() -> (w84:dbl)
            n230 = Divide(x=w83, y=10.0) -> (x/y=w81:dbl)
            n231 = Greater?(x=w83, y=150.0) -> (0:w85:bool)
            n232 = Less?(x=w84, y=w81) -> (x < y?=w86:bool)
            n233 = local read "Power Output"() -> (w97:bool)
            n234 = And(x=w85, y=w86) -> (x .and. y?=w79:bool)
            n235 = local read "time"() -> (w94:dbl)
            n236 = local write "VISA resource name"(w105) -> ()
            n237 = local write "PSU error message"(w104) -> ()
            n238 = call <vilib>:"High Resolution Relative Seconds.vi"() -> ("relative seconds"=w95:dbl)
            n239 = Not(x=w97) -> (.not. x?=w80:bool)
            n240 = Bundle(w91, w90) -> (w99:cluster{dbl[], dbl[]})  [unwired: 1 in]
            n241 = local write "I(V) Graph"(w99) -> ()
            n242 = Or(x=w79, y=w80) -> (x .or. y?=w78:bool)
            n243 = Subtract(x=w95, y=w94) -> (x-y=w93:dbl)
            n244 = Build Array (concatenate)(w96, w93) -> (w92:dbl[])
            n245 = Bundle(w92, w90) -> (w89:cluster{dbl[], dbl[]})  [unwired: 1 in]
            n246 = local write "V(t)"(w89) -> ()
            n247 = Bundle(w92, w91) -> (w88:cluster{dbl[], dbl[]})  [unwired: 1 in]
            n248 = local write "I(t)"(w88) -> ()
          }
          n249 = local read "Filename"() -> (w66:string)
          n250 = Equal?(x="", y=w66) -> (x = y?=w64:bool)
          n251 = case shown="False" w64 {
            tunnel: w68 -> [w77 _]
            tunnel: w67 -> [w76 _]
            tunnel: w66 -> [w72 _]
            frame False {
              n252 = Build Array(w77, w76) -> (w75:dbl[][])
              n253 = Transpose 2D Array(2D array=w75) -> (transposed array=w74:dbl[][])
              n254 = call "WriteHeaderAndDataFile.vi"("filename"=w72, "Array"=w74, "Header"="Current (A)     Voltage (V)") -> ()
            }
            frame True {
            }
          }
        }
        frame #2 {
          # "Turn off PSU after measurements"
          n255 = local read "VISA resource name"() -> (w333:refnum<visa-resource-name>)
          n256 = local read "PSU error message"() -> (w332:errorcluster)
          n257 = VISA Write(VISA resource name=w333, write buffer="OUTP OFF", error in (no error)=w332) -> (VISA resource name out=w330:refnum<visa-resource-name>, error out=w329:errorcluster)  [unwired: 1 out]
          n258 = call "Close.vi"("error in (no error)"=w329, "VISA resource name"=w330) -> ("error out"=w328:errorcluster)  [unwired: 9 in]
          n259 = local write "PSU error message"(w328) -> ()
        }
      }
    }
  }
